vi "Dialog_spectr (SubVI).vi"() -> ()   [LabVIEW 2017]
uses:
  <vilib>/Analysis/4window.llb/windowTd.ctl
  Control_EU/AScan3.ctl
  <vilib>/measure/maspectr.llb/FFT Spectrum (Mag-Phase) for N Chan.vi
  Global_SNK3_HF.vi
  <vilib>/measure/NI_MAPro.lvlib
  <vilib>/Analysis/NI_AALPro.lvlib
panel:
  in  "AScan":T1
  in  "averaging":T2={"averaging mode"=enum."RMS averaging", "weighting mode"=enum."Exponential", "number of averages"=16} {"number of averages" min=1}
  in  "window":T3=1 items=["Rectangle"=0, "Hanning"=1, "Hamming"=2, "Blackman-Harris"=3, "Exact Blackman"=4, "Blackman"=5, "Flat Top"=6, "4 Term B-Harris "=7, "7 Term B-Harris"=8, "Low Sidelobe"=9, "Blackman Nuttall"=11, "Triangle"=30, "Bartlett-Hanning"=31, "Bohman"=32, "Parzen"=33, "Welch"=34, "Kaiser"=60, "Dolph-Chebyshev"=61, "Gaussian"=62]
  in  "dB":bool
  out "spectrum":cluster{"f0":dbl, "df":dbl, "magnitude":dbl[]}[](graph)=[{"f0"=0.0, "df"=49999.99999999999, "magnitude"=[0.009570402801989028, 1.1145988206786688, 2.099197531478026, 2.0197125274878256, 1.384124712324977, 0.9095779916480808, 0.6327236728323555, 0.44877847466880644, 0.3328494604687887, 0.25125410738824977, 0.20071363200895143, 0.17236554850409203, 0.18961893976079208, 0.23025542012990818, 0.08733419690734098, 0.16945843994504375, 0.10017284761090013, 0.08270514361135832, 0.07026633457307933, 0.07418964799596102, 0.05372117588087633, 0.05946499548172138, 0.049049368195951785, 0.050543788109402146, 0.044158841793182815, 0.042026208163654905, 0.03420636086838049, 0.031177545589619982, 0.0351030507078099, 0.025245398489777842, 0.0313371175735453, 0.028587161755929815, 0.02290983648822749, 0.029044591008553777, 0.01975639592748353, 0.023553715923246753, 0.025857325199385623, 0.01940329433717839, 0.031007810004861445, 0.024828290881232992, 0.025332903912414505, 0.021258763536226483, 0.027731111100886826, 0.024230485263696113, 0.02017176018177204, 0.02624686248118884, 0.022582787627767505, 0.0200235889445197, 0.020692930861508762, 0.023583915755430118, 0.021027200096049387, 0.023767338829136956, 0.026453421951273287, 0.023948778604670675, 0.02137049575710814, 0.025036500813449235, 0.02585270092543584, 0.025174679759712607, 0.030561707476376036, 0.029720880997500376, 0.02882417440011868, 0.026689509761550705, 0.02744048990538022, 0.023945643466111808, 0.02696285413299574, 0.02660945885425799, 0.025009348432219556, 0.024416917705855173, 0.02793478552958608, 0.024458911131190756, 0.02927605282331396, 0.019989728296821295, 0.02667411146586328, 0.023406319991204464, 0.02273127316208246, 0.025893372299175443, 0.027371404001108865, 0.027175245052207163, 0.02194850309397964, 0.028284238577995165, 0.0318313022841646, 0.022601927598573813, 0.019368050233495287, 0.018903782528370515, 0.017753675587752635, 0.020525477562869952, 0.023140873008896518, 0.026707514253994334, 0.01925673851482763, 0.020540214761260864, 0.02548498480904517, 0.021936916439902414, 0.026508216421486673, 0.022221329812236335, 0.018870545524074436, 0.020005660398300564, 0.024285593598141857, 0.024464043557209412, 0.022607807816654082, 0.02183058508649068, 0.023833810436431367, 0.021654759778127215, 0.022084876867694826, 0.022041591946658598, 0.027500452136798952, 0.032089197815329054, 0.024656294553454854, 0.020712424137031917, 0.021737572675466357, 0.02115661316677075, 0.021652185926049745, 0.021792989578248812, 0.019803581585042564, 0.021212344190718112, 0.021048175499144568, 0.01834427619091851, 0.02252008779109783, 0.023463782638494867, 0.01973863706907999, 0.018953110261499137, 0.019418666049077726, 0.018034257574919298, 0.019010909494170235, 0.021368306620788806, 0.023562598615649726, 0.02544381085345141, 0.020356206453773344, 0.017393271012861033, 0.018046235645249167, 0.017044933498316303, 0.016763176466868555, 0.015108373076498295, 0.01747026163015727, 0.022656840658868384, 0.025103978154197664, 0.02448956420379529, 0.021094878907018513, 0.018017927916657555, 0.01949030517284597, 0.020717957823766703, 0.021233873495477684, 0.015941870238178207, 0.016212935391187608, 0.01698112314662892, 0.01608707911332905, 0.020828207936696742, 0.018473993096554037, 0.02054571487668001, 0.02286675643182689, 0.02160178904477323, 0.018811591738985636, 0.02079665283041097, 0.020575485082892343, 0.018358268286147915, 0.018945323935043737, 0.01636035379462932, 0.01719634200077758, 0.01545662361890321, 0.015338679148117347, 0.014394647195423113, 0.015114221790905866, 0.017554494672533498, 0.015174521358137037, 0.017242529420087648, 0.0218818082625245, 0.018304504134805208, 0.01640160190597529, 0.02081761310429843, 0.01786931421134815, 0.015067559062204753, 0.0192092968891698, 0.020253045598918974, 0.01675140742066832, 0.014701735975818654, 0.015106517597198476, 0.01579345191196456, 0.017835347667407693, 0.01652991252257055, 0.014451120588374366, 0.014466267940694997, 0.016503997435347337, 0.017514897799851346, 0.016524042503071924, 0.01624405830829541, 0.014576106836718384, 0.014528097710660035, 0.014238213463744206, 0.014834751571630556, 0.01530264761769489, 0.014292156177519395, 0.01356305941883994, 0.01779315077218456, 0.02029316843439108, 0.020197758404786288, 0.012726598289496396, 0.01508661707650156, 0.012540600498894555, 0.014547469477108447, 0.011270698960494688, 0.014757647910774335, 0.015026905734414077, 0.014979676608323007, 0.015674561313874156, 0.011582952798043195, 0.01281244325678687, 0.012825071440289234, 0.013185502790433774, 0.015170744198971235, 0.013118173507164113, 0.014553886621809526, 0.012663031363962114, 0.01312633728321765, 0.012804538701633944, 0.01405996230199971, 0.012584938237469482, 0.009402057773006574, 0.013080241161554804, 0.014398532810455961, 0.01560561708450041, 0.013451014227053413, 0.011773938989314819, 0.010374002002429545, 0.012711864611507981, 0.010662568528439949, 0.009952764112292886, 0.011041231125722284, 0.012037315259747688, 0.013724855535009902, 0.013592570889310374, 0.014952570609098343, 0.012328600374180154, 0.010431506162941591, 0.011405350435853072, 0.009224029196094753, 0.009957779343517853, 0.011608974138896645, 0.010770734409538735, 0.011833877155029425, 0.01127540003475986, 0.00956617842699061, 0.010075808316633635, 0.009864051682825099, 0.008705324596707364, 0.008727859232532408, 0.011591441783522774, 0.01239210053435623, 0.009144133946272545, 0.007834673017962108, 0.008313077518913626, 0.009616421486975696, 0.008674572888702912, 0.009314731944595082, 0.00987988070306082, 0.010136772220072225, 0.009230710444680547, 0.007443576861341017, 0.00760806222427338, 0.008769514125877998, 0.008537355290568736, 0.010042245359087458, 0.009023223782872371, 0.00673078203319742, 0.006834557149320207, 0.007460717472521303, 0.008040453683135378, 0.009429178776435974, 0.007510163277904474, 0.006813397449608024, 0.008941948801401284, 0.009730404106227322, 0.009174648918768971, 0.008022430605117958, 0.008424581353917684, 0.00749827242386753, 0.0059805725052981895, 0.0061639914945693835, 0.00634092314209063, 0.006808954993775319, 0.006811969131919291, 0.006636034931115964, 0.00692590361721146, 0.006096878681662024, 0.00563014785171432, 0.006212478959156243, 0.006691325977656149, 0.005432877150957887, 0.006311109549854385, 0.005125973912418523, 0.007816563141865915, 0.008205027392522896, 0.005698512133000745, 0.00518170644389982, 0.004509393830716246, 0.0043923937738255805, 0.006357844798250102, 0.0060404946373425064, 0.00656781358308477, 0.004938194931585116, 0.0052492436280852164, 0.006123766764547694, 0.0061226452151916105, 0.006019579044977614, 0.004474831046335469, 0.004852418457232893, 0.004929111335491809, 0.004591601773954245, 0.004635756328459637, 0.004738966123000512, 0.003856704967385384, 0.0031026650923064642, 0.0037920621056316984, 0.003673144430356548, 0.003901074005426476, 0.004125144276071376, 0.004132727994204674, 0.0032121590992622642, 0.00279369158088327, 0.00431269105763806, 0.005237466417082352, 0.004062835292731981, 0.0033657026275961035, 0.00418754544578938, 0.005103083032490537, 0.004297788027933915, 0.0038903568487547568, 0.0037831936908660946, 0.00431502777778049, 0.003987431508137257, 0.0038432543653509456, 0.003507265583167809, 0.0035921332029030303, 0.003729889452303599, 0.0035830821851443487, 0.0026931423915531705, 0.0030606642369380398, 0.003248035338979637, 0.0030232441638439445, 0.002973201468042902, 0.0036385351347875262, 0.003849797051608863, 0.0026821795366011557, 0.003224277248189308, 0.0027353634305024147, 0.001957730685666126, 0.002723046530544468, 0.002200178271221791, 0.0031788410557011667, 0.003689640267690925, 0.0026686972881866636, 0.0020681121674429015, 0.0021068093521828574, 0.0021806689700414462, 0.00291351419127389, 0.002988719081448778, 0.0029164029639758312, 0.0025693063233710573, 0.0020285988614200828, 0.0019283299160713352, 0.0016522740427826416, 0.0019530692240721291, 0.0022110853528767216, 0.001908665709548311, 0.001971939988873016, 0.0022448474423690085, 0.002171059113762283, 0.0017694948349920743, 0.0017507729673331997, 0.0020411247896679223, 0.0018624386404451573, 0.0016546982235234732, 0.0017012941398146097, 0.0016599031507372325, 0.001776898985757592, 0.001339238649972658, 0.001265723078231505, 0.0013975236046927927, 0.0014854862025372845, 0.0013934943210214463, 0.001449299434435507, 0.0016068937894007937, 0.0014192876660632377, 0.0013849763209510353, 0.0011232548713332605, 0.0009503898069726815, 0.0010352928517822352, 0.0010910955452447064, 0.0010490923343264341, 0.000979198223208966, 0.001071701488126968, 0.0012425318703010342, 0.0009162659828829774, 0.0010343966073644247, 0.0011465609867719756, 0.0009733512124846575, 0.0009615153614048867, 0.0008214078429582976, 0.0007275779367713006, 0.000833701530699879, 0.0005914779278686768, 0.0006547645798882388, 0.000825879313069261, 0.0005799932193941874, 0.0005844663089209437, 0.000730702617453865, 0.0006004262111439593, 0.0005281828813768407, 0.0004766783814596537, 0.0004390046878886272, 0.0005072823728957131, 0.00038887748611656615, 0.0005246558644336697, 0.0004237454284607491, 0.0004846455019959116, 0.00038092247209813035, 0.000345399649298286, 0.00045086093130043106, 0.0004530753589951481, 0.00041627535523857485, 0.00039433191956607237, 0.0003376705328277122, 0.00033398135852876653, 0.0003092134083241773, 0.0002560972429120827, 0.00028205301478411793, 0.00031984450047810255, 0.00024373461474682734, 0.000227943915947789, 0.00022722089828452593, 0.0002331832377475103, 0.00019974209220837056, 0.00019136925878356805, 0.00020651793153921854, 0.00014524329388610065, 0.00018028629382063377, 0.0001538725869960289, 0.0001646691954493728, 0.00011729614251206292, 0.00013200598702946137, 0.00011341856772551211, 9.825771507368206e-05, 0.00010100945790399977, 9.580667327123526e-05, 7.733042510327136e-05, 6.472883720106998e-05, 8.768371271682528e-05, 8.882802538462494e-05, 0.0001030486352360837, 6.753537405979789e-05, 7.385536421943597e-05, 7.118378462428873e-05, 6.520335722135961e-05, 4.3223801547973193e-05, 5.7955308290734646e-05, 5.419522104464845e-05, 4.056756052932771e-05, 5.166090950162183e-05, 3.565949206933345e-05, 3.930009682303647e-05, 4.457327169889828e-05, 3.120150416076682e-05, 3.197984037565442e-05, 3.0839867631384856e-05, 2.457417540650372e-05, 2.8442647060644194e-05, 2.5188077938371733e-05, 2.0075261828238798e-05, 1.9711697922977205e-05, 2.1251348766976508e-05, 1.7033492848379882e-05, 1.89684780164676e-05, 1.4417312049796038e-05, 1.3928555311996393e-05, 1.299683312496495e-05, 1.0299519927753502e-05, 1.0686936634154616e-05, 8.537416521875065e-06, 9.759164300666474e-06, 6.010440045753248e-06, 6.0380864413589794e-06, 6.09413076765543e-06, 5.117415814047459e-06, 3.737177960627587e-06, 4.113835704507036e-06, 3.255456209015391e-06, 2.8994166796621733e-06, 3.0930441629502894e-06, 2.7466689787547053e-06, 2.8207305403792647e-06, 2.7774548666952252e-06, 2.5380664027923305e-06, 2.587220519937837e-06, 2.354872000633125e-06, 2.340097366253538e-06, 2.1208203293556933e-06, 1.937229225809131e-06, 1.7210815244965155e-06, 1.4723725711714136e-06, 1.2553410413655826e-06, 1.0225369026772575e-06, 8.63015859578035e-07]}, ...(80 in all)]
  in  "ScaleOrdinate":T4(ring)=enum."Вольты" caption="Ось ординат"
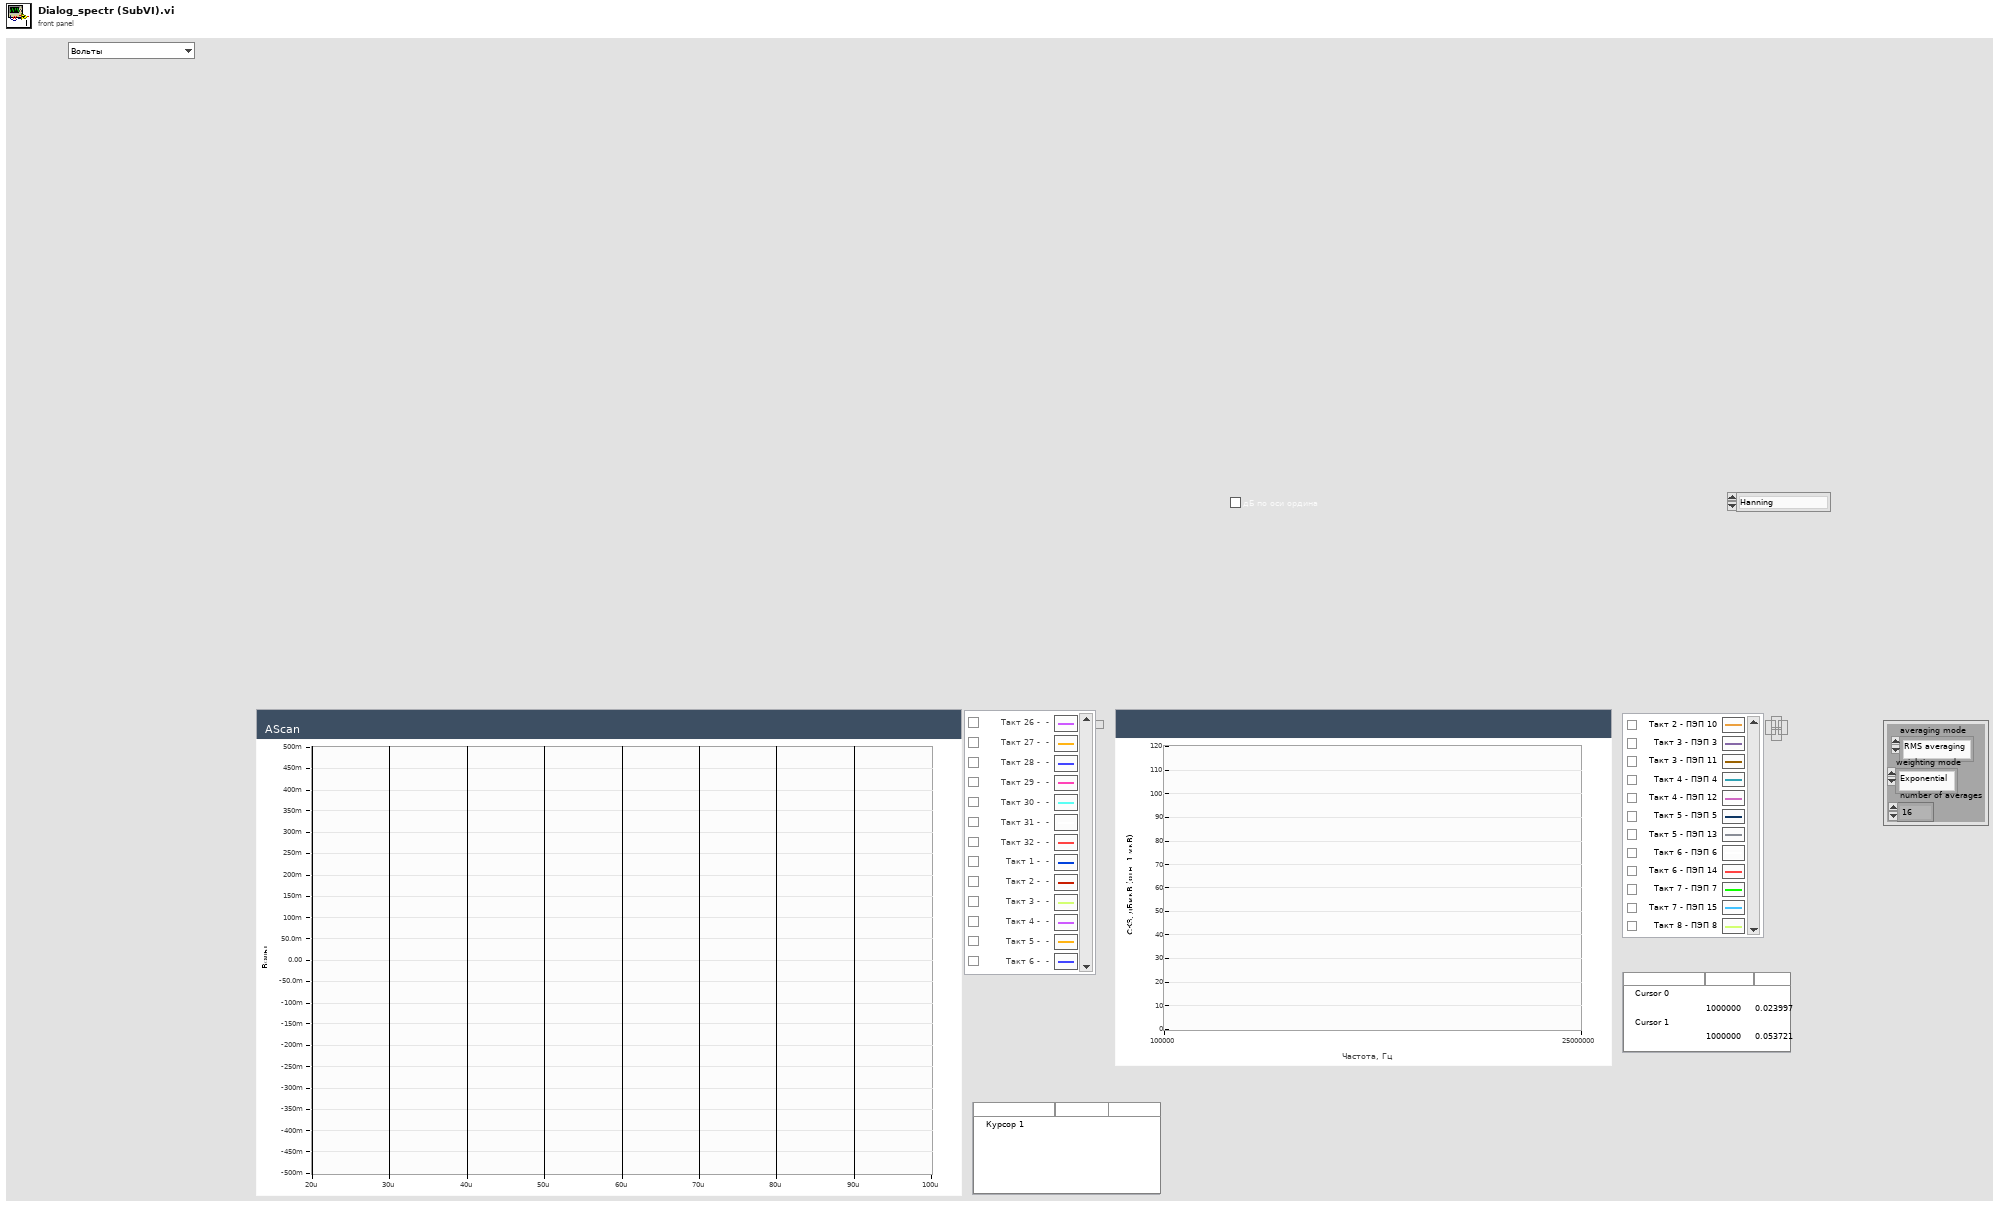
[diagram p1: front panel]
types:
  T1 = typedef "AScan3.ctl" = cluster{"f0":dbl, "df":dbl, "magnitude":dbl[]}[]
  T2 = cluster{"averaging mode":enum16{"No averaging", "Vector averaging", "RMS averaging", "Peak hold"}, "weighting mode":enum16{"Linear", "Exponential"}, "number of averages":u32}
  T3 = typedef "NI_AALPro.lvlib/windowTd.ctl" = u32
  T4 = enum16{"Отсчеты АЦП (±32767)", "Проценты", "Вольты", "дБмкВ (отн. 1 мкВ)", "Отсчеты АЦП (±1)"}
  T5 = cluster{"dB On (F)":bool, "unwrap phase (F)":bool, "convert to degree (F)":bool}
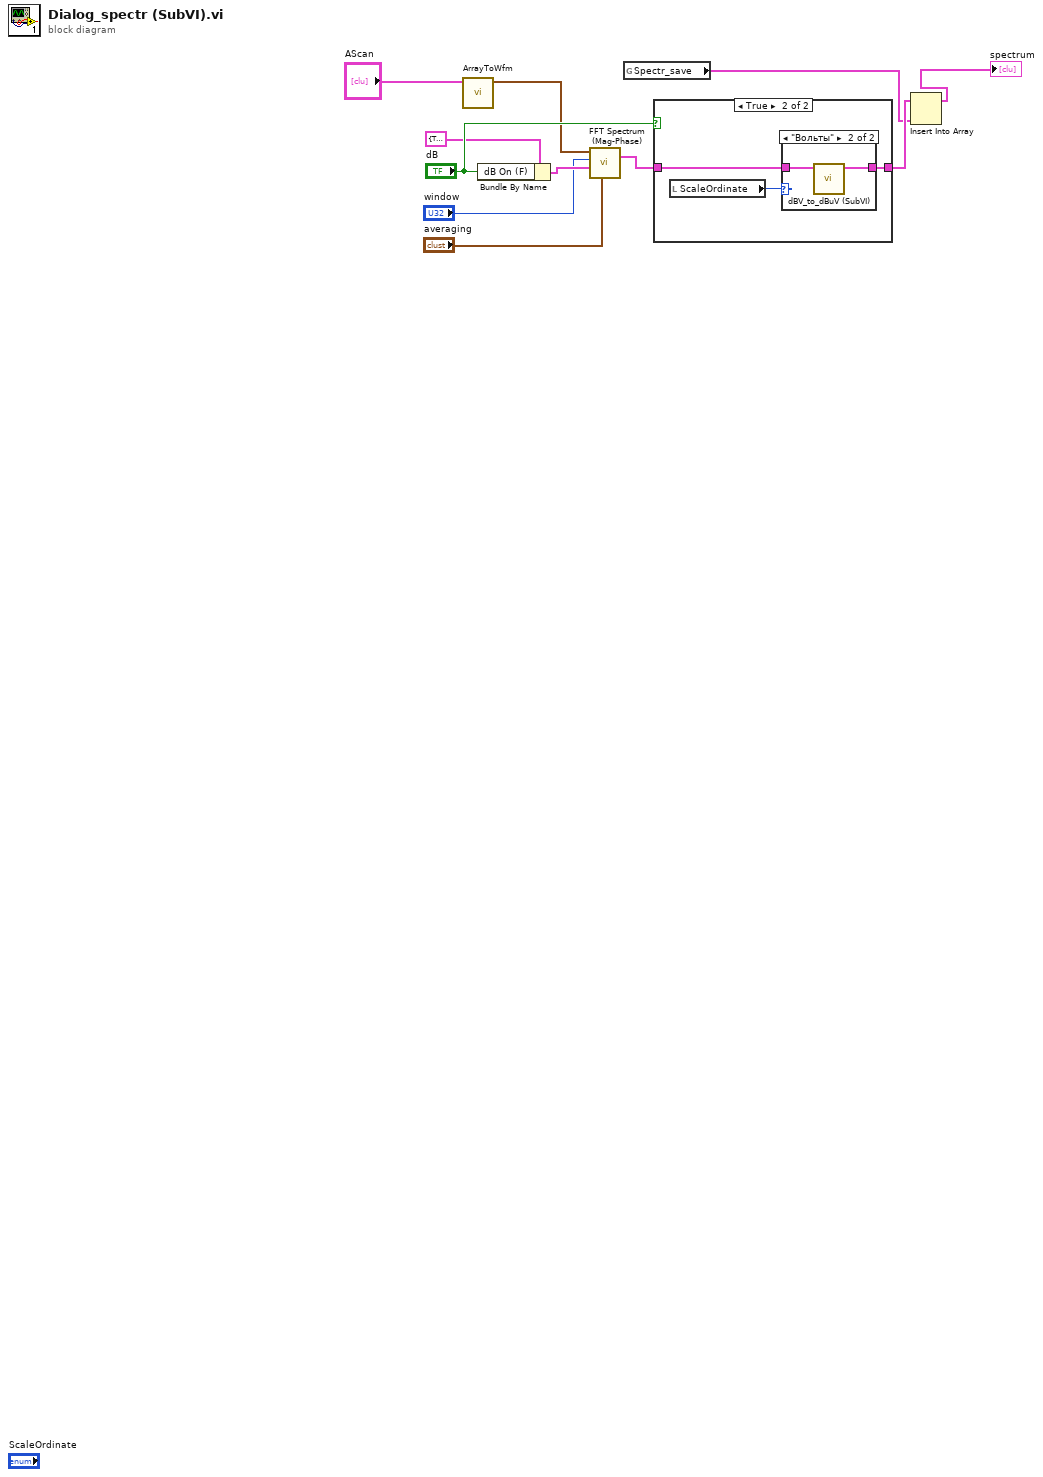
[diagram p0: block diagram]
diagram:
  n1 = call "ArrayToWfm.vi"("Magnitude"="AScan") -> ("time signals"=w4:waveform(dbl)[])  [unwired: 10 in]
  n2 = Bundle By Name(cluster=T5 {"dB On (F)"=TRUE, "unwrap phase (F)"=FALSE, "convert to degree (F)"=FALSE} ("view"), "dB On (F)"="dB") -> (w8:T5)
  n3 = call-poly <vilib>:"FFT Spectrum (Mag-Phase).vi"("averaging parameters"="averaging", "view"=w8, "window"="window", "time signals"=w4) -> ("magnitudes"=w10:cluster{"f0":dbl, "df":dbl, "magnitude":dbl[]}[])  [unwired: 3 in, 4 out]
  n4 = global read "Global_SNK3_HF.vi" "Spectr_save"() -> (w1:cluster{"f0":dbl, "df":dbl, "magnitude":dbl[]}[])
  n5 = case shown="True" "dB" {
    tunnel: w10 -> [w12 w13]
    tunnel: [w12 w15] -> w3
    frame False {
    }
    frame True {
      n6 = local read "ScaleOrdinate"() -> (w14:T4)
      n7 = case shown="\"Вольты\"" w14 {
        tunnel: w13 -> [w16 w18]
        tunnel: [w16 w17] -> w15
        frame "Отсчеты АЦП (±32767)", Default {
        }
        frame "Вольты" {
          n8 = call "dBV_to_dBuV (SubVI).vi"("magnitudes"=w18) -> ("Array"=w17:cluster{"f0":dbl, "df":dbl, "magnitude":dbl[]}[])  [unwired: 10 in]
        }
      }
    }
  }
  n9 = Insert Into Array(array=w3, new element=w1) -> (→"spectrum":cluster{"f0":dbl, "df":dbl, "magnitude":dbl[]}[])  [unwired: 1 in]
